vi "Start.vi"(8 "error in":errorcluster, 11 "NEO480 in":refnum<class "Virtual NEO480.lvclass">) -> (0 "error out":errorcluster, 3 "NEO480 out":refnum<class "Virtual NEO480.lvclass">)   [LabVIEW 2024, in "Virtual NEO480.lvclass"]
uses:
  Virtual NEO480.lvclass
  Virtual NEO480.lvclass/Virtual NEO480.ctl
  Source/DBC Communicator/DBC Communicator.lvclass
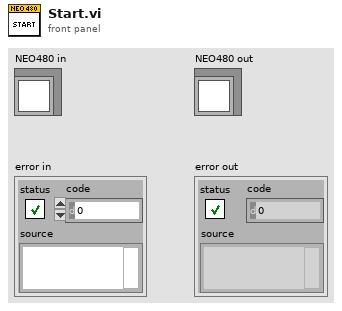
[diagram p1: front panel]
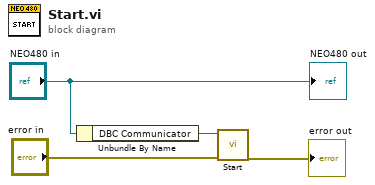
[diagram p0: block diagram]
diagram:
  n1 = Unbundle By Name("NEO480 in") -> ("DBC Communicator"=w2:refnum<class "DBC Communicator.lvclass">)
  n2 = call-dynamic "Start.vi"("Error In"="error in", "Communicator in"=w2) -> ("Error Out"=→"error out":errorcluster)  [unwired: 8 in, 1 out]
  "NEO480 out" <- "NEO480 in"
